vi "getSubArray_Bella.vi"(7 "element":string, 8 "error in (no error)":errorcluster, 11 "Array IN":string[][](array[string])) -> (0 "error out":errorcluster, 3 "Array out":dbl[](array[numeric]))   [LabVIEW 2020]
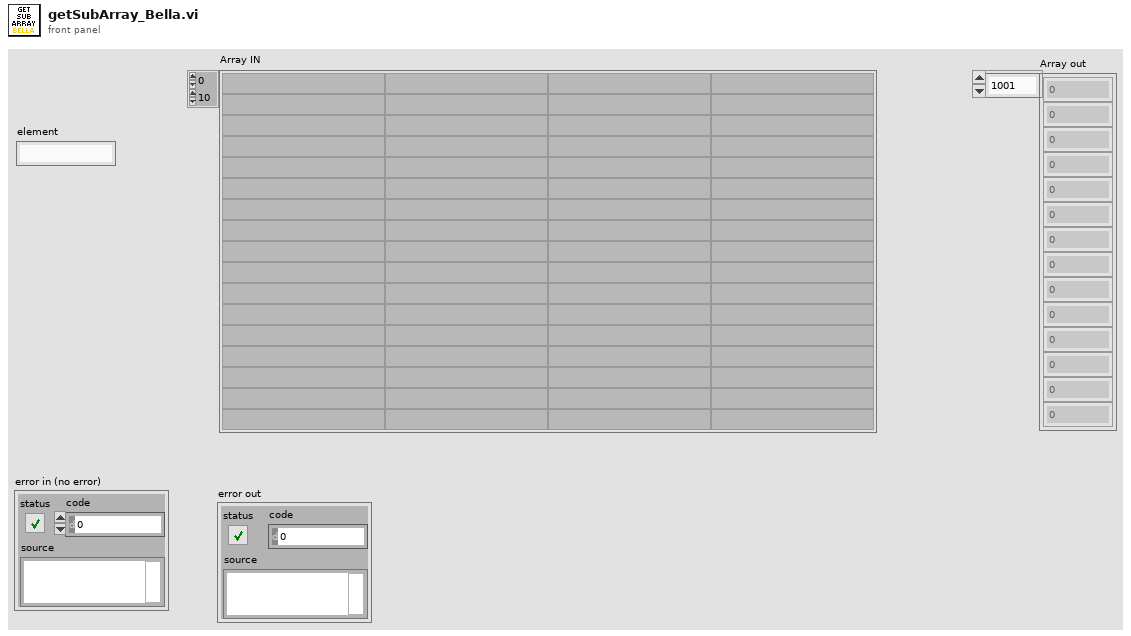
[diagram p1: front panel]
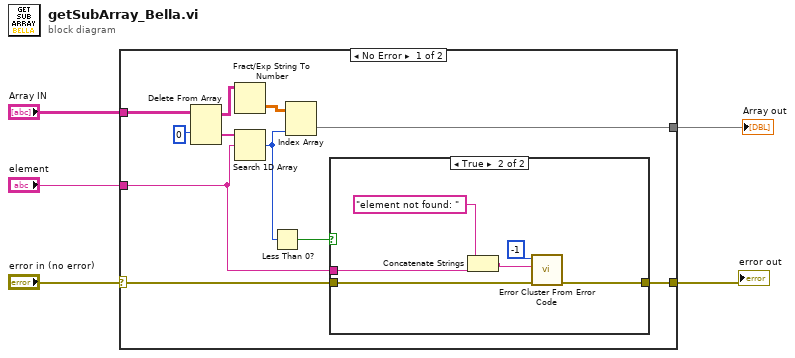
[diagram p0: block diagram]
diagram:
  n1 = case shown="No Error" "error in (no error)" {
    selector: "error in (no error)" -> [w6 w24]
    tunnel: [w16 _] -> w5
    tunnel: "element" -> [w8 _]
    tunnel: "Array IN" -> [w13 _]
    tunnel: [w7 w24] -> w1
    frame No Error {
      n2 = Delete From Array(array=w13, index (row)=0) -> (deleted portion=w12:string[], array with subset deleted=w15:string[][])  [unwired: 2 in]
      n3 = Fract/Exp String To Number(string=w15) -> (number=w11:dbl[][])  [unwired: 3 in, 1 out]
      n4 = Search 1D Array(1D array=w12, element=w8) -> (index of element=w10:i32)  [unwired: 1 in]
      n5 = Less Than 0?(x=w10) -> (x < 0?=w9:bool)
      n6 = Index Array(array=w11, index (col)=w10) -> (element=w16:dbl[])  [unwired: 1 in]
      n7 = case shown="True" w9 {
        tunnel: w8 -> [_ w21]
        tunnel: [w17 w19] -> w7
        tunnel: w6 -> [w17 w18]
        frame False {
        }
        frame True {
          n8 = Concatenate Strings("element not found: ", w21) -> (w20:string)
          n9 = call <vilib>:"Error Cluster From Error Code.vi"("error in (no error)"=w18, "error message (\"\")"=w20, "error code (0)"=-1) -> ("error out"=w19:errorcluster)  [unwired: 6 in]
        }
      }
    }
    frame Error {
    }
  }
  "Array out" <- w5
  "error out" <- w1
